vi "Stop.vi"(8 "error in (no error)":errorcluster, 9 "Channel Data (DBLs Only)":T1={"Inputs"={"Data to Server"=1.0}, "Outputs"={"Data from Server"=0.0}}, 10 "Real-Time System Data":T2, 11 "Configuration Data":T3={"Timeout (ms)"=100, "Server IP"="localhost", "Port"=6340}) -> (0 "error out":errorcluster)   [LabVIEW 2013, in "TCPIP Custom Device.lvlib"]
uses:
  TCPIP Custom Device.lvlib
  Configuration Data.ctl
  Real-Time System Data.ctl
  Channel Data.ctl
panel:
  # "Controls"
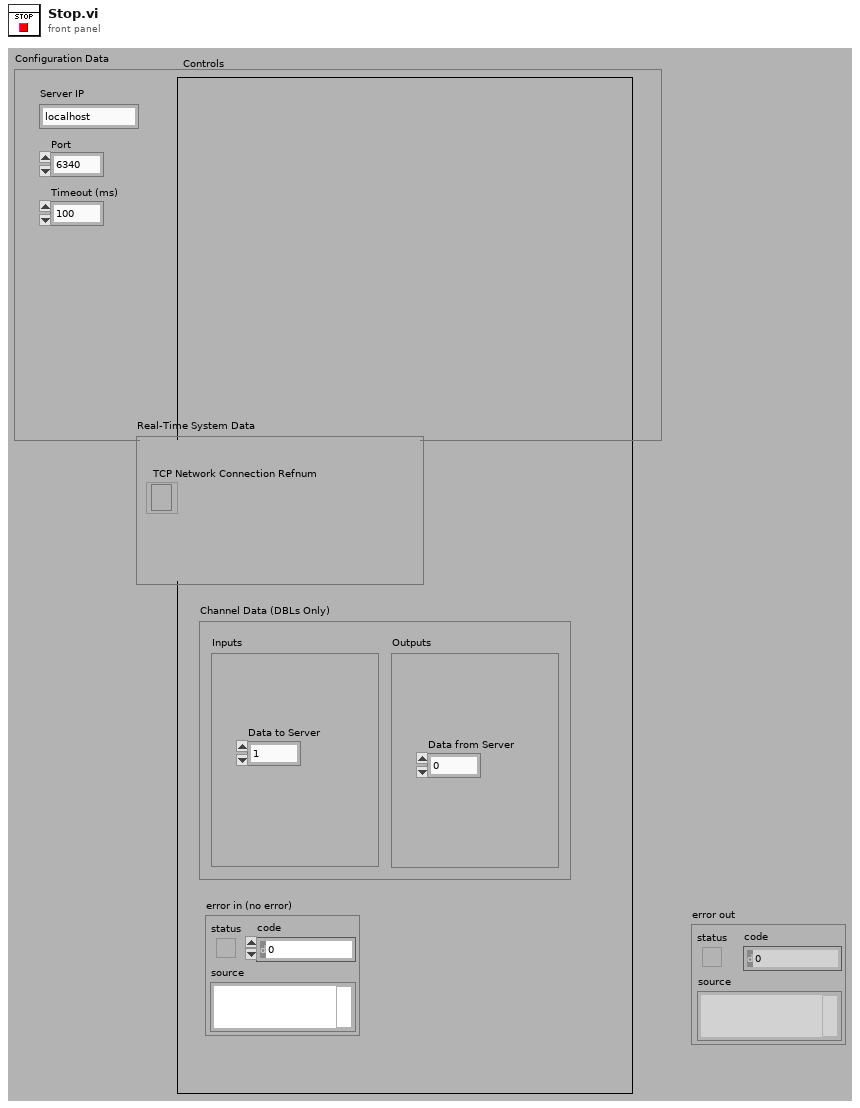
[diagram p1: front panel]
types:
  T1 = typedef "TCPIP Custom Device.lvlib/Channel Data.ctl" = cluster{"Inputs":cluster{"Data to Server":dbl}, "Outputs":cluster{"Data from Server":dbl}}
  T2 = typedef "TCPIP Custom Device.lvlib/Real-Time System Data.ctl" = cluster{"TCP Network Connection Refnum":refnum<k5>}
  T3 = typedef "TCPIP Custom Device.lvlib/Configuration Data.ctl" = cluster{"Timeout (ms)":i32, "Server IP":string, "Port":i32}
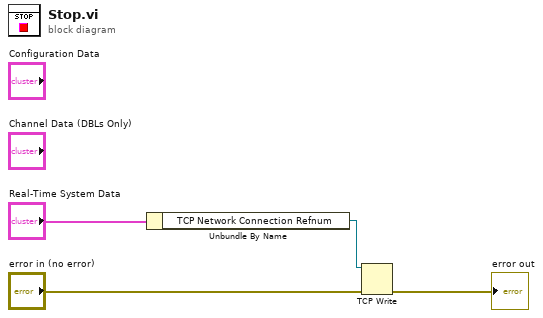
[diagram p0: block diagram]
diagram:
  n1 = Unbundle By Name("Real-Time System Data") -> ("TCP Network Connection Refnum"=w4:refnum<k5>)
  n2 = TCP Write(connection ID=w4, error in (no error)="error in (no error)") -> (error out=→"error out":errorcluster)  [unwired: 1 in, 3 out]
